vi "Read.vi"(8 "error in (no error)":errorcluster, 11 "Boolean in":refnum<class "Boolean.lvclass">) -> (0 "error out":errorcluster, 2 "Boolean":bool, 3 "Boolean out":refnum<class "Boolean.lvclass">)   [LabVIEW 2020, in "Data.lvlib" / "Boolean.lvclass"]
doc: "Read boolean."
uses:
  Boolean.lvclass
  Boolean.lvclass/Boolean.ctl
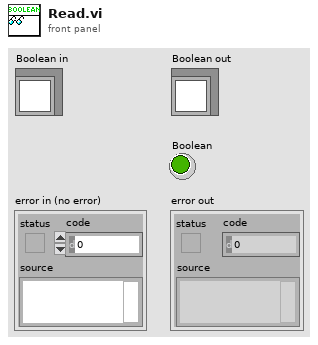
[diagram p1: front panel]
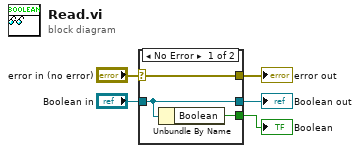
[diagram p0: block diagram]
diagram:
  n1 = case shown="No Error" "error in (no error)" {
    selector: "error in (no error)" -> [w8 w9]
    tunnel: [w8 w9] -> w4
    tunnel: [w7 w10] -> w2
    tunnel: "Boolean in" -> [w7 w10]
    tunnel: [w6 _] -> w1
    frame No Error {
      n2 = Unbundle By Name(w7) -> ("Boolean"=w6:bool)
    }
    frame Error {
    }
  }
  "error out" <- w4
  "Boolean out" <- w2
  "Boolean" <- w1
